vi "StripNonAscii.vi"(1 "Incoming String":string) -> (0 "Outgoing String":string)   [LabVIEW 2013]
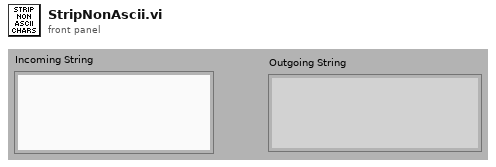
[diagram p1: front panel]
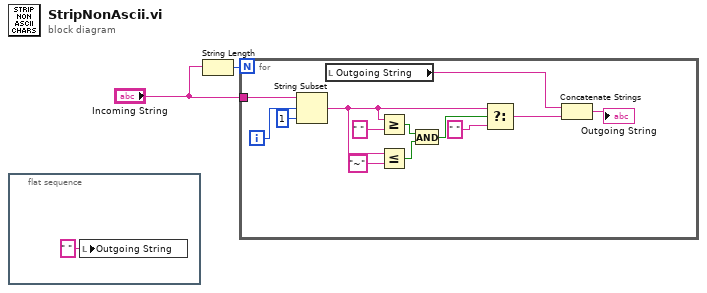
[diagram p0: block diagram]
diagram:
  n1 = flat-sequence {
    frame #0 {
      n2 = local write "Outgoing String"(" " ("Outgoing String")) -> ()
    }
  }
  n3 = String Length(string="Incoming String") -> (length=w2:i32)
  n4 = for {
    N: w2 -> [_]
    tunnel: "Incoming String" -> [w15]
    i -> [w14]
    n5 = String Subset(string=w15, offset (0)=w14, length (rest)=1 ("length (rest)")) -> (substring=w8:string)
    n6 = local read "Outgoing String"() -> (w12:string)
    n7 = Greater Or Equal?(x=w8, y=" ") -> (x >= y?=w6:bool)
    n8 = Less Or Equal?(x=w8, y="~") -> (x <= y?=w5:bool)
    n9 = And(x=w6, y=w5) -> (x .and. y?=w4:bool)
    n10 = Select(t=w8, s=w4, f=" ") -> (s? t:f=w11:string)
    n11 = Concatenate Strings(w12, w11) -> (→"Outgoing String":string)
  }
